vi "TPM with correction version 10-1-1 imaging_Min_20180112.vi"() -> ()   [LabVIEW 2018]
uses:
  Casao LabVIEW SDK 1.0.5/Haso/Data Haso/Wavefront parameters.ctl
  Casao LabVIEW SDK 1.0.5/Casao/Casao/Loop prefs.ctl
  Casao LabVIEW SDK 1.0.5/Haso/Data Haso/DataHaso.ctl
  <vilib>/Utility/file.llb/Read From Spreadsheet File (DBL).vi
  <vilib>/Utility/file.llb/Write To Spreadsheet File (DBL).vi
panel:
  in  "galvo phase":dbl=89.0
  out "output path":path
  out "Model Coefficients (µm) after":sgl[](array[numeric])
  out "Model Coefficients (µm) before":sgl[](array[numeric])
  in  "stop":bool
  out "Slice now":dbl
  in  "Iteration #":u16(ring)=1 items=["1"=1, "2"=2, "3"=3, "4"=4, "5"=5]
  in  "AO Exp Time":dbl(ring)=0.5 items=["0.2s"=0.2, "0.5s"=0.5, "1.0s"=1.0, "1.5s"=1.5]
  out "after correction":T1
  in  "Filter y tilt":bool=TRUE
  in  "Filter x tilt":bool=TRUE
  in  "Curvature filter":bool=TRUE
  out "PV":dbl
  out "RMS":dbl
  in  "Matrix path":path=path "C:/Documents and Settings/User/Desktop/zw/20160113 200nm bead command matrix.aomc"
  in  "Offset path":path=path "C:/Documents and Settings/User/Desktop/zw/2016-02-09 system resolution/100nm bead correction.dat"
  out "Camera image":u32[][](graph)
  out "RMS":dbl
  out "PV":dbl
  out "before correction":T1
  in  "Curvature filter":bool=TRUE
  in  "Filter y tilt":bool=TRUE
  in  "Filter x tilt":bool=TRUE
  out "after correction":dbl[][](graph) caption="Wavefront"
  out "before correction":dbl[][](graph) caption="Wavefront"
  in  "EMCCD ImExp Time (s)":dbl(ring)=0.5 items=["0.2"=0.2, "0.5"=0.5, "1.0"=1.0, "4.0"=4.0, "8.0"=8.0]
  in  "Step size(um)":dbl
  in  "Laser Power%(0-100)":dbl=10.0
  in  "Slices #":dbl=1.0
  in  "Average Frame #":dbl=10.0
  in  "Correction":bool
  # "OFF"
  # "ON"
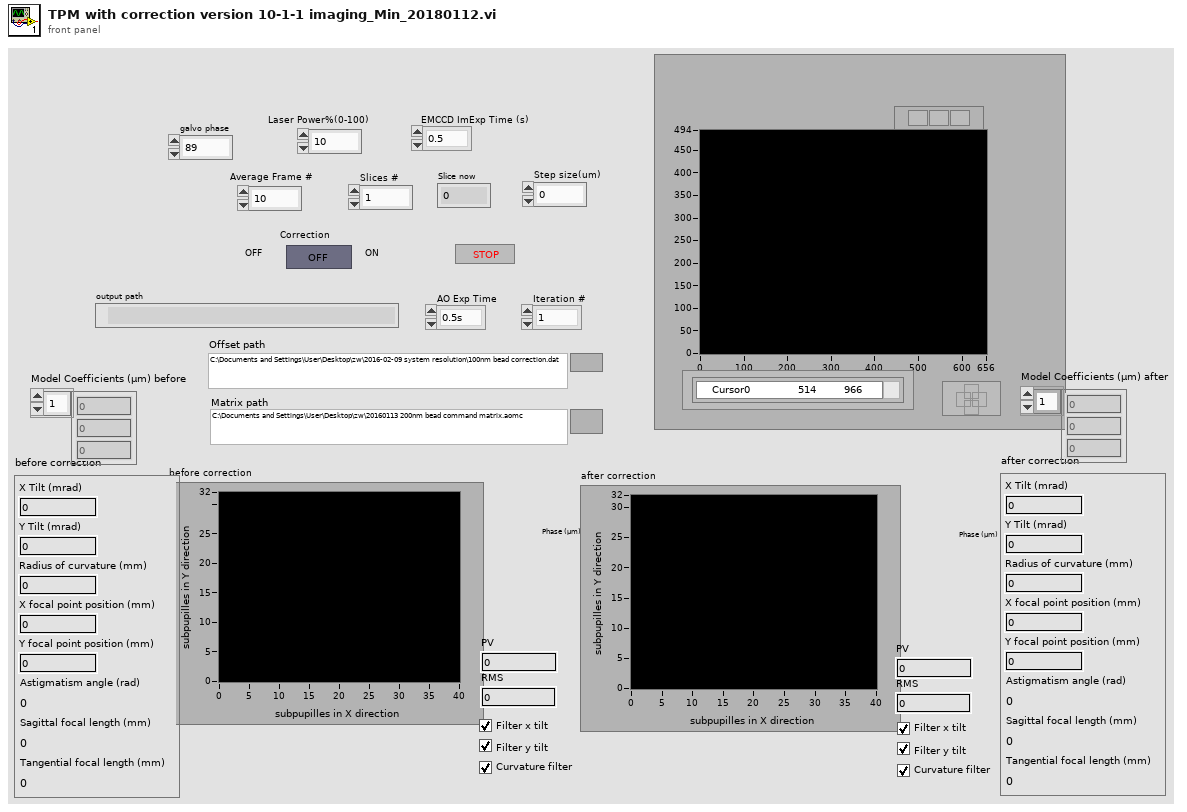
[diagram p1: front panel]
types:
  T1 = typedef "Wavefront parameters.ctl" = cluster{"X Tilt (mrad)":sgl, "Y Tilt (mrad)":sgl, "Radius of curvature (mm)":sgl, "X focal point position (mm)":sgl, "Y focal point position (mm)":sgl, "Astigmatism angle (rad)":sgl, "Sagittal focal length (mm)":sgl, "Tangential focal length (mm)":sgl}
  T2 = typedef "Loop prefs.ctl" = cluster{"Filter tilt on measurement (closed loop)":bool, "Correction gain (closed loop)":sgl, "Limit of subapertures off in CGP (%)":sgl, "Limit of saturated actuators (%)":sgl}
  T3 = cluster{"Filtre tilt X":bool, "Filtre tilt Y":bool, "Filtre courbure":bool}
  T4 = typedef "DataHaso.ctl" = i32
  T5 = cluster{"Measurement":T4, "Target":T4, "Manual target":T4}
  T6 = cluster{"Target for tilt":T4, "Target for focus":T4, "Target for all other aberrations":T4}
  T7 = typedef "Camera.ctl" = i32
  T8 = typedef "PhaseModul.ctl" = i32
  T9 = typedef "Haso.ctl" = i32
  T10 = typedef "Casao.ctl" = i32
  T11 = typedef "Image Compat.ctl" = cluster{"Signed/unsigned":bool, "Number of bits":T12, "Internal object id":i32, "Internal data id":i32}
  T12 = typedef "Data alignment enum.ctl" = enum16{"8", "16", "32"}
  T13 = typedef "Reconstruction prefs.ctl" = cluster{"Reconstruction type":enum16{"Modal", "Zonal"}, "Polynomial type":enum16{"Zernike", "Legendre"}, "Modal reconstruction prefs":T14, "Zonal reconstruction prefs":T17}
  T14 = typedef "Modal reconstruction prefs.ctl" = cluster{"Number of coefficients":u32, "Filtered coefficients":u32[], "RMS Zernike normalization":bool, "Matrix inversion method":u16, "Add zonal residual to modal fit ":bool, "Detection prefs":T15}
  T15 = typedef "PupilDetectionPrefs.ctl" = cluster{"Automatic pupil detection":bool, "Central occultation pupil":bool, "Semi-automatic pupil detection (find radius)":bool, "Semi-automatic pupil detection (find center)":bool, "Automatic pupil detection mode":enum16{"Contained", "Containing"}, "Start coordinates":cluster{"Pupil center (Zernike)":T16, "Pupil radius (Zernike)":sgl, "Pupil center (Legendre)":T16, "Pupil halfsize (Legendre)":T16}}
  T16 = typedef "Point2Df.ctl" = cluster{"X":sgl, "Y":sgl}
  T17 = typedef "Zonal reconstruction prefs.ctl" = cluster{"Number of weak iterations":u16, "Number of max iterations":u32, "Residual limit":sgl}
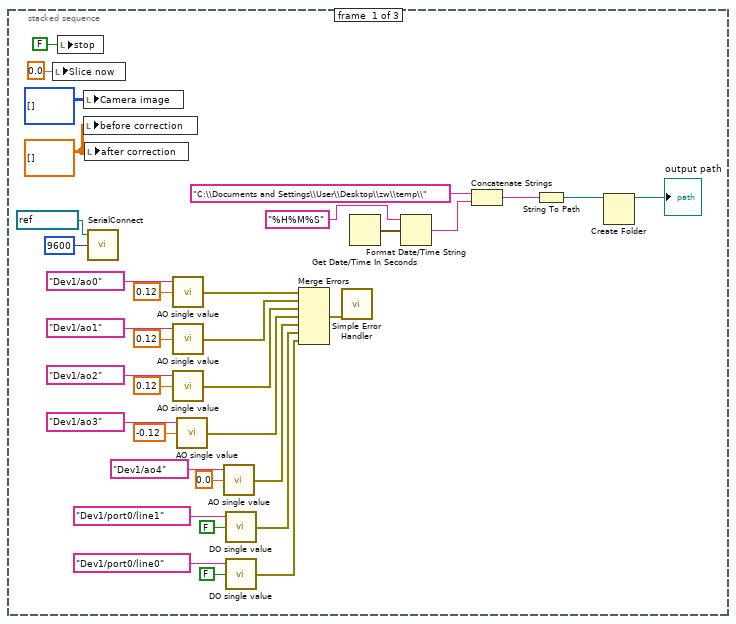
[diagram p2: hidden frame]
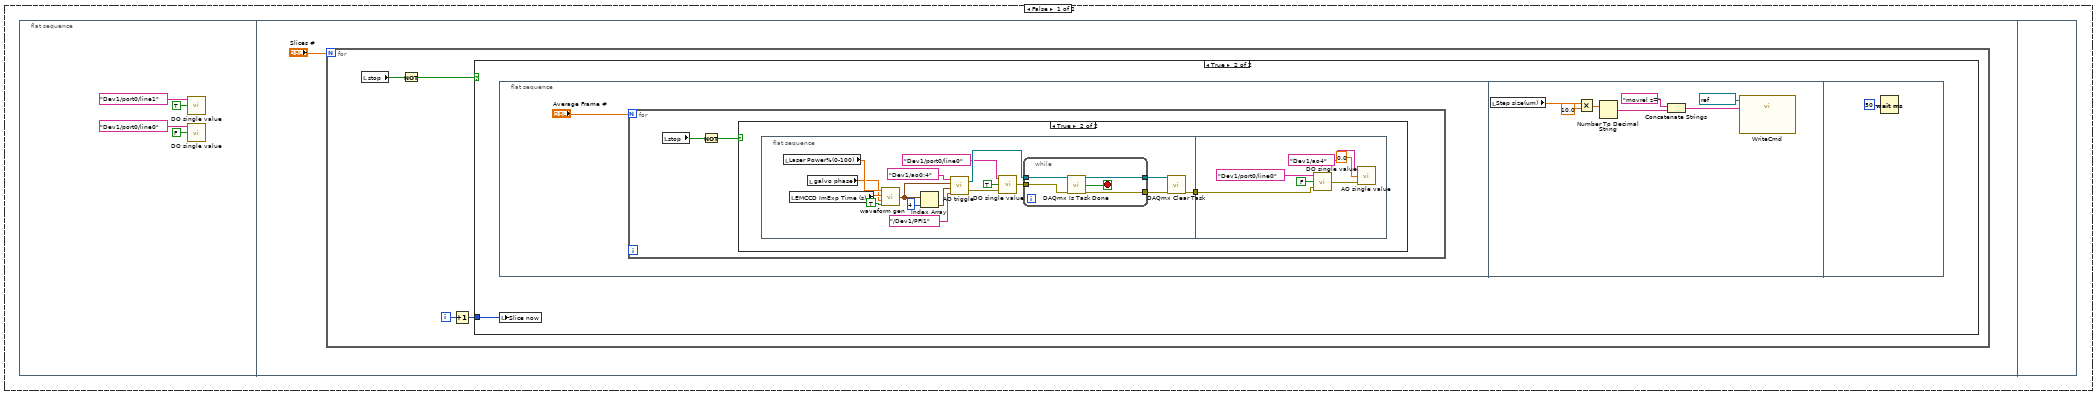
[diagram p3: hidden frame]
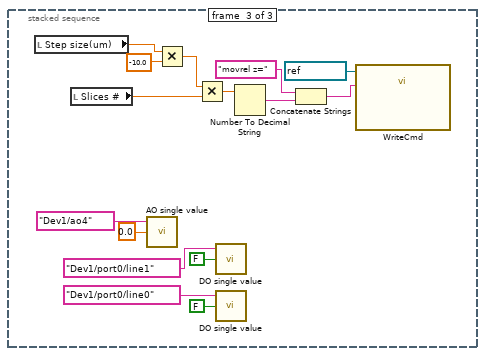
[diagram p10: hidden frame]
diagram:
  n1 = stacked-sequence {
    frame #0 {
      w34 = dbl[][] [] ("before correction")
      n2 = local write "Slice now"(0.0 ("Slice now")) -> ()
      n3 = local write "stop"(FALSE ("stop")) -> ()
      n4 = local write "Camera image"(u32[][] [] ("Camera image")) -> ()
      n5 = local write "before correction"(w34) -> ()
      n6 = local write "after correction"(w34) -> ()
      n7 = call "SerialConnect.vi"("baud rate (9600)"=u32 9600, "VISA resource name"=refnum<visa-resource-name> "COM1") -> ()  [unwired: 1 in, 3 out]
      n8 = call "AO single value.vi"("data"=0.12, "physical channels"=tag "Dev1/ao0") -> ("error out"=w17:errorcluster)  [unwired: 1 in]
      n9 = call "AO single value.vi"("data"=0.12, "physical channels"=tag "Dev1/ao1") -> ("error out"=w16:errorcluster)  [unwired: 1 in]
      n10 = call "AO single value.vi"("data"=0.12, "physical channels"=tag "Dev1/ao2") -> ("error out"=w15:errorcluster)  [unwired: 1 in]
      n11 = call "AO single value.vi"("data"=-0.12, "physical channels"=tag "Dev1/ao3") -> ("error out"=w14:errorcluster)  [unwired: 1 in]
      n12 = call "AO single value.vi"("data"=0.0, "physical channels"=tag "Dev1/ao4") -> ("error out"=w13:errorcluster)  [unwired: 1 in]
      n13 = call "DO single value.vi"("data"=FALSE, "lines"=tag "Dev1/port0/line1") -> ("error out"=w12:errorcluster)  [unwired: 1 in]
      n14 = call "DO single value.vi"("data"=FALSE, "lines"=tag "Dev1/port0/line0") -> ("error out"=w10:errorcluster)  [unwired: 1 in]
      n15 = Merge Errors(w17, w16, w15, w14, w13, w12, w10) -> (w11:errorcluster)
      n16 = call <vilib>:"Simple Error Handler.vi"("error in (no error)"=w11) -> ()  [unwired: 4 in, 5 out]
      n17 = Get Date/Time In Seconds() -> (seconds since 1Jan1904=w2:timestamp)
      n18 = Format Date/Time String(time format string (%c)="%H%M%S", seconds (now)=w2) -> (date/time string=w5:string)  [unwired: 1 in]
      n19 = Concatenate Strings("C:\\Documents and Settings\\User\\Desktop\\zw\\temp\\" ("string"), w5) -> (w6:string)
      n20 = String To Path(string=w6) -> (path=w7:path)
      n21 = Create Folder(path (use dialog)=w7) -> (created path=→"output path":path)  [unwired: 2 in, 2 out]
    }
    frame #1 {
      n22 = case shown="True" "Correction" {
        frame False {
          n23 = flat-sequence {
            frame #0 {
              n24 = call "DO single value.vi"("data"=TRUE, "lines"=tag "Dev1/port0/line1") -> ()  [unwired: 1 in, 1 out]
              n25 = call "DO single value.vi"("data"=FALSE, "lines"=tag "Dev1/port0/line0") -> ()  [unwired: 1 in, 1 out]
            }
            frame #1 {
              n26 = for {
                N: "Slices #" -> [_]
                i -> [w45]
                n27 = local read "stop"() -> (w43:bool)
                n28 = Not(x=w43) -> (.not. x?=w42:bool)
                n29 = Increment(x=w45) -> (x+1=w44:i32)
                n30 = case shown="True" w42 {
                  tunnel: w44 -> [_ w46]
                  frame False {
                  }
                  frame True {
                    n31 = local write "Slice now"(w46) -> ()
                    n32 = flat-sequence {
                      frame #0 {
                        n33 = for {
                          N: "Average Frame #" -> [_]
                          n34 = local read "stop"() -> (w48:bool)
                          n35 = Not(x=w48) -> (.not. x?=w49:bool)
                          n36 = case shown="True" w49 {
                            frame False {
                            }
                            frame True {
                              n37 = flat-sequence {
                                tunnel: [w52] -> w50
                                tunnel: w50 -> [w74]
                                frame #0 {
                                n38 = local read "Laser Power%(0-100)"() -> (w63:dbl)
                                n39 = local read "EMCCD ImExp Time (s)"() -> (w62:dbl)
                                n40 = local read "galvo phase"() -> (w51:dbl)
                                n41 = call "waveform gen.vi"("Boolean"=TRUE, "galvo phase"=w51, "Exposure Time (s)"=w62, "Laser Power%(0-100)"=w63) -> ("waveform"=w60:waveform(dbl)[])
                                n42 = Index Array(array=w60, index=4) -> (element=w61:waveform(dbl))
                                n43 = call "AO triggle.vi"("physical channels"=tag "Dev1/ao0:4", "data"=w60, "waveform"=w61, "trig source"=tag "/Dev1/PFI1") -> ("task out"=w57:refnum<k21>, "error out"=w54:errorcluster)  [unwired: 1 in]
                                n44 = call "DO single value.vi"("error in"=w54, "data"=TRUE, "lines"=tag "Dev1/port0/line0") -> ("error out"=w53:errorcluster)
                                n45 = while {
                                tunnel: [w72] -> w66
                                tunnel: [w71] -> w65
                                tunnel: w57 -> [w69]
                                tunnel: w53 -> [w68]
                                stop <- w70 stop-if-true
                                n46 = call <vilib>:"DAQmx Is Task Done.vi"("task/channels in"=w69, "error in"=w68) -> ("task out"=w72:refnum<k21>, "task done?"=w70:bool, "error out"=w71:errorcluster)  [unwired: 11 in]
                                }
                                n47 = call <vilib>:"DAQmx Clear Task.vi"("task in"=w66, "error in"=w65) -> ("error out"=w52:errorcluster)  [unwired: 13 in]
                                }
                                frame #1 {
                                n48 = call "DO single value.vi"("error in"=w74, "data"=FALSE, "lines"=tag "Dev1/port0/line0") -> ("error out"=w73:errorcluster)
                                n49 = call "AO single value.vi"("error in"=w73, "data"=0.0, "physical channels"=tag "Dev1/ao4") -> ()  [unwired: 1 out]
                                }
                              }
                            }
                          }
                        }
                      }
                      frame #1 {
                        n50 = local read "Step size(um)"() -> (w79:dbl)
                        n51 = Multiply(x=w79, y=10.0) -> (x*y=w81:dbl)
                        n52 = Number To Decimal String(number=w81) -> (decimal integer string=w84:string)  [unwired: 1 in]
                        n53 = Concatenate Strings("movrel z=", w84) -> (w83:string)
                        n54 = call "WriteCmd.vi"("Command"=w83, "VISA resource name"=refnum<visa-resource-name> "COM1") -> ()  [unwired: 1 in, 1 out]
                      }
                      frame #2 {
                        n55 = Wait (ms)(milliseconds to wait=u32 50) -> ()  [unwired: 1 out]
                      }
                    }
                  }
                }
              }
            }
            frame #2 {
            }
          }
        }
        frame True {
          n56 = flat-sequence {
            tunnel: [w102] -> w94
            tunnel: [w104] -> w93
            tunnel: [w103] -> w92
            tunnel: [w102] -> w91
            tunnel: [w101] -> w90
            tunnel: [w100] -> w88
            tunnel: [w95] -> w87
            tunnel: w94 -> [w123]
            tunnel: w93 -> [w122]
            tunnel: w92 -> [w121]
            tunnel: w91 -> [w118]
            tunnel: w90 -> [w117]
            tunnel: [w120] -> w89
            tunnel: w88 -> [w114]
            tunnel: w87 -> [w115]
            tunnel: w89 -> [w639]
            frame #0 {
              n57 = call "AO single value.vi"("data"=0.0, "physical channels"=tag "Dev1/ao4") -> ()  [unwired: 1 in, 1 out]
              n58 = local read "AO Exp Time"() -> (w105:dbl)
              n59 = call-poly <vilib>:"Read From Spreadsheet File.vi"("format (%.3f)"="%.8f", "file path (dialog if empty)"="Offset path") -> ("first row"=w95:dbl[])  [unwired: 5 in, 4 out]
              n60 = call "DO single value.vi"("data"=TRUE, "lines"=tag "Dev1/port0/line1") -> ()  [unwired: 1 in, 1 out]
              n61 = call "DO single value.vi"("data"=FALSE, "lines"=tag "Dev1/port0/line0") -> ()  [unwired: 1 in, 1 out]
              n62 = call "AO init.vi"("Exposure duration specified (s)"=w105, "Commands in"=w95, "Matrix path"="Matrix path") -> ("error out"=w102:errorcluster, "Camera"=w104:T7, "Mirror"=w100:T8, "Haso"=w103:T9, "Casao"=w101:T10)  [unwired: 3 in, 1 out]
            }
            frame #1 {
              n63 = call "Casao Set Preferences.vi"("error in (no error)"=w118, "Loop preferences"=T2 {"Filter tilt on measurement (closed loop)"=FALSE, "Correction gain (closed loop)"=0.75, "Limit of subapertures off in CGP (%)"=0.0, "Limit of saturated actuators (%)"=0.0}, "Casao"=w117) -> ("error out"=w112:errorcluster, "Casao (dup)"=w116:T10)  [unwired: 3 in]
              n64 = local read "Slices #"() -> (w124:dbl)
              n65 = call "PhaseModul apply command.vi"("error in (no error)"=w112, "Commands in"=w115, "Mirror"=w114) -> ("error out"=w111:errorcluster, "Mirror (dup)"=w113:T8)  [unwired: 2 in, 1 out]
              n66 = for {
                N: w124 -> [_]
                tunnel: w123 -> [w138]
                tunnel: w122 -> [w137]
                tunnel: w121 -> [w136]
                tunnel: w111 -> [w126]
                tunnel: [w135] -> w120
                tunnel: w113 -> [w127]
                tunnel: w116 -> [w134]
                tunnel: w115 -> [w125]
                i -> [w130]
                n67 = local read "stop"() -> (w132:bool)
                n68 = Increment(x=w130) -> (x+1=w133:i32)
                n69 = local write "Slice now"(w133) -> ()
                n70 = Not(x=w132) -> (.not. x?=w131:bool)
                n71 = case shown="True" w131 {
                  tunnel: w138 -> [_ w147]
                  tunnel: w137 -> [_ w146]
                  tunnel: w136 -> [_ w145]
                  tunnel: w126 -> [_ w144]
                  tunnel: [w139 w141] -> w135
                  tunnel: w127 -> [_ w143]
                  tunnel: w134 -> [w139 w142]
                  tunnel: w125 -> [_ w140]
                  frame False {
                  }
                  frame True {
                    n72 = flat-sequence {
                      tunnel: w147 -> [w187]
                      tunnel: w146 -> [w186]
                      tunnel: w145 -> [w185]
                      tunnel: w144 -> [w181]
                      tunnel: w143 -> [w172]
                      tunnel: w142 -> [w170]
                      tunnel: [w149] -> w141
                      tunnel: w140 -> [w148]
                      frame #0 {
                        n73 = flat-sequence {
                          tunnel: w170 -> [w190]
                          tunnel: w172 -> [w191]
                          tunnel: w181 -> [w192]
                          tunnel: w185 -> [w193]
                          tunnel: w186 -> [w194]
                          tunnel: w187 -> [w195]
                          tunnel: [w195] -> w155
                          tunnel: [w194] -> w154
                          tunnel: [w193] -> w153
                          tunnel: [w192] -> w152
                          tunnel: [w191] -> w151
                          tunnel: [w190] -> w150
                          tunnel: [w202] -> w161
                          tunnel: [w201] -> w160
                          tunnel: [w200] -> w159
                          tunnel: [w199] -> w158
                          tunnel: [w198] -> w157
                          tunnel: [w197] -> w156
                          tunnel: w155 -> [w202]
                          tunnel: w154 -> [w201]
                          tunnel: w153 -> [w200]
                          tunnel: w152 -> [w199]
                          tunnel: w151 -> [w198]
                          tunnel: w150 -> [w197]
                          tunnel: [w231] -> w184
                          tunnel: [w240] -> w183
                          tunnel: [w239] -> w182
                          tunnel: [w235] -> w180
                          tunnel: [w236] -> w179
                          tunnel: [w233] -> w173
                          tunnel: w161 -> [w232]
                          tunnel: w160 -> [w240]
                          tunnel: w159 -> [w239]
                          tunnel: w158 -> [w236]
                          tunnel: w157 -> [w234]
                          tunnel: w156 -> [w235]
                          tunnel: w148 -> [w230]
                          tunnel: w184 -> [w282]
                          tunnel: w183 -> [w281]
                          tunnel: w182 -> [w280]
                          tunnel: w180 -> [w279]
                          tunnel: w179 -> [w278]
                          tunnel: [w258] -> w178
                          tunnel: [w257] -> w177
                          tunnel: [w253] -> w176
                          tunnel: [w251] -> w175
                          tunnel: [w249] -> w174
                          tunnel: w173 -> [w244]
                          tunnel: [w243] -> w171
                          tunnel: [w241] -> w163
                          tunnel: w178 -> [w425]
                          tunnel: w177 -> [w424]
                          tunnel: w176 -> [w422]
                          tunnel: w175 -> [w421]
                          tunnel: w174 -> [w420]
                          tunnel: [w419] -> w169
                          tunnel: w171 -> [w418]
                          tunnel: [w417] -> w168
                          tunnel: [w416] -> w167
                          tunnel: [w415] -> w166
                          tunnel: [w414] -> w165
                          tunnel: [w413] -> w164
                          tunnel: w163 -> [w412]
                          tunnel: [w412] -> w162
                          tunnel: w169 -> [w604]
                          tunnel: w168 -> [w623]
                          tunnel: w167 -> [w622]
                          tunnel: w166 -> [w621]
                          tunnel: w165 -> [w611]
                          tunnel: w164 -> [w612]
                          tunnel: w162 -> [w610]
                          tunnel: [w604] -> w149
                          frame #0 {
                            n74 = call "AO single value.vi"("data"=-5.0, "physical channels"=tag "Dev1/ao5") -> ()  [unwired: 1 in, 1 out]
                          }
                          frame #1 {
                            n75 = local read "Average Frame #"() -> (w196:dbl)
                            n76 = for {
                              N: w196 -> [_]
                              n77 = local read "stop"() -> (w203:bool)
                              n78 = Not(x=w203) -> (.not. x?=w204:bool)
                              n79 = case shown="True" w204 {
                                frame False {
                                }
                                frame True {
                                n80 = flat-sequence {
                                frame #0 {
                                n81 = local read "Laser Power%(0-100)"() -> (w216:dbl)
                                n82 = local read "EMCCD ImExp Time (s)"() -> (w215:dbl)
                                n83 = call "waveform gen.vi"("Boolean"=TRUE, "galvo phase"="galvo phase", "Exposure Time (s)"=w215, "Laser Power%(0-100)"=w216) -> ("waveform"=w213:waveform(dbl)[])
                                n84 = Index Array(array=w213, index=4) -> (element=w214:waveform(dbl))
                                n85 = call "AO triggle.vi"("physical channels"=tag "Dev1/ao0:4", "data"=w213, "waveform"=w214, "trig source"=tag "/Dev1/PFI1") -> ("task out"=w210:refnum<k21>, "error out"=w207:errorcluster)  [unwired: 1 in]
                                n86 = call "DO single value.vi"("error in"=w207, "data"=TRUE, "lines"=tag "Dev1/port0/line0") -> ("error out"=w206:errorcluster)
                                n87 = while {
                                tunnel: [w225] -> w219
                                tunnel: [w224] -> w218
                                tunnel: w210 -> [w222]
                                tunnel: w206 -> [w221]
                                stop <- w223 stop-if-true
                                n88 = call <vilib>:"DAQmx Is Task Done.vi"("task/channels in"=w222, "error in"=w221) -> ("task out"=w225:refnum<k21>, "task done?"=w223:bool, "error out"=w224:errorcluster)  [unwired: 11 in]
                                }
                                n89 = call <vilib>:"DAQmx Clear Task.vi"("task in"=w219, "error in"=w218) -> ()  [unwired: 13 in, 1 out]
                                }
                                frame #1 {
                                n90 = call "AO single value.vi"("data"=0.0, "physical channels"=tag "Dev1/ao4") -> ()  [unwired: 1 in, 1 out]
                                n91 = call "DO single value.vi"("data"=FALSE, "lines"=tag "Dev1/port0/line0") -> ()  [unwired: 1 in, 1 out]
                                }
                                }
                                }
                              }
                            }
                          }
                          frame #2 {
                            n92 = call "PhaseModul apply command.vi"("error in (no error)"=w232, "Commands in"=w230, "Mirror"=w234) -> ("error out"=w231:errorcluster, "Mirror (dup)"=w233:T8)  [unwired: 2 in, 1 out]
                            n93 = call "AO single value.vi"("data"=1.0, "physical channels"=tag "Dev1/ao5") -> ()  [unwired: 1 in, 1 out]
                          }
                          frame #3 {
                            n94 = flat-sequence {
                              tunnel: [w291] -> w277
                              tunnel: [w290] -> w276
                              tunnel: [w289] -> w275
                              tunnel: [w288] -> w274
                              tunnel: [w287] -> w273
                              tunnel: w280 -> [w289]
                              tunnel: w281 -> [w290]
                              tunnel: w282 -> [w291]
                              tunnel: [w286] -> w272
                              tunnel: w279 -> [w286]
                              tunnel: [w285] -> w271
                              tunnel: w278 -> [w285]
                              tunnel: [w284] -> w245
                              tunnel: w244 -> [w284]
                              tunnel: w277 -> [w307]
                              tunnel: w276 -> [w308]
                              tunnel: w275 -> [w309]
                              tunnel: [w309] -> w270
                              tunnel: [w306] -> w269
                              tunnel: [w305] -> w268
                              tunnel: [w304] -> w267
                              tunnel: w274 -> [w304]
                              tunnel: [w303] -> w266
                              tunnel: w273 -> [w303]
                              tunnel: [w302] -> w265
                              tunnel: w272 -> [w302]
                              tunnel: [w301] -> w264
                              tunnel: w271 -> [w301]
                              tunnel: [w300] -> w246
                              tunnel: w245 -> [w300]
                              tunnel: w270 -> [w321]
                              tunnel: [w321] -> w261
                              tunnel: [w320] -> w262
                              tunnel: w269 -> [w320]
                              tunnel: [w319] -> w263
                              tunnel: w268 -> [w319]
                              tunnel: w267 -> [w314]
                              tunnel: w266 -> [w313]
                              tunnel: [w312] -> w260
                              tunnel: w265 -> [w312]
                              tunnel: [w311] -> w259
                              tunnel: w264 -> [w311]
                              tunnel: [w310] -> w247
                              tunnel: w246 -> [w310]
                              tunnel: w263 -> [w404]
                              tunnel: w262 -> [w364]
                              tunnel: w261 -> [w365]
                              tunnel: w260 -> [w390]
                              tunnel: w259 -> [w389]
                              tunnel: [w368] -> w256
                              tunnel: [w367] -> w255
                              tunnel: [w366] -> w254
                              tunnel: [w365] -> w252
                              tunnel: [w364] -> w250
                              tunnel: [w363] -> w248
                              tunnel: w247 -> [w362]
                              tunnel: [w362] -> w242
                              tunnel: [w336] -> w241
                              tunnel: [w410] -> w257
                              tunnel: [w411] -> w258
                              tunnel: w256 -> [w411]
                              tunnel: w255 -> [w410]
                              tunnel: w254 -> [w409]
                              tunnel: [w408] -> w253
                              tunnel: w252 -> [w408]
                              tunnel: [w407] -> w251
                              tunnel: w250 -> [w407]
                              tunnel: [w406] -> w249
                              tunnel: w248 -> [w406]
                              tunnel: [w405] -> w243
                              tunnel: w242 -> [w405]
                              frame #0 {
                                n95 = local read "Laser Power%(0-100)"() -> (w297:dbl)
                                n96 = local read "AO Exp Time"() -> (w296:dbl)
                                n97 = local read "galvo phase"() -> (w283:dbl)
                                n98 = call "waveform gen.vi"("Boolean"=FALSE, "galvo phase"=w283, "Exposure Time (s)"=w296, "Laser Power%(0-100)"=w297) -> ("waveform"=w295:waveform(dbl)[])
                                n99 = Index Array(array=w295, index=4) -> (element=w294:waveform(dbl))
                                n100 = call "AO triggle.vi"("physical channels"=tag "Dev1/ao0:4", "data"=w295, "waveform"=w294, "trig source"=tag "/Dev1/PFI1") -> ("task out"=w288:refnum<k21>, "error out"=w287:errorcluster)  [unwired: 1 in]
                              }
                              frame #1 {
                                n101 = call "Camera Start.vi"("error in (no error)"=w307, "camera"=w308) -> ("error out"=w305:errorcluster, "camera (dup)"=w306:T7)  [unwired: 4 in]
                              }
                              frame #2 {
                                n102 = while {
                                tunnel: [w327] -> w316
                                tunnel: [w326] -> w315
                                tunnel: w314 -> [w324]
                                tunnel: w313 -> [w323]
                                i -> [w322]
                                stop <- w325 stop-if-true
                                n103 = local write "Slice now"(w322) -> ()
                                n104 = call <vilib>:"DAQmx Is Task Done.vi"("task/channels in"=w324, "error in"=w323) -> ("task out"=w327:refnum<k21>, "task done?"=w325:bool, "error out"=w326:errorcluster)  [unwired: 11 in]
                                }
                                n105 = call "DO single value.vi"("data"=TRUE, "lines"=tag "Dev1/port0/line0") -> ()  [unwired: 1 in, 1 out]
                                n106 = call <vilib>:"DAQmx Clear Task.vi"("task in"=w316, "error in"=w315) -> ()  [unwired: 13 in, 1 out]
                              }
                              frame #3 {
                                n107 = call "Camera Get image.vi"("error in (no error)"=w404, "camera"=w364) -> ("error out"=w386:errorcluster, "Image"=w387:T11, "camera (dup)"=w388:T7)  [unwired: 3 in]
                                n108 = call "Camera Stop.vi"("error in (no error)"=w386, "camera"=w388) -> ()  [unwired: 4 in, 2 out]
                                n109 = call "Image get data.vi"("error in (no error)"=w386, "Image Compat"=w387) -> ("error out"=w376:errorcluster, "Array"=w385:u32[][], "Image Compat (dup)"=w375:T11)  [unwired: 3 in]
                                n110 = call "AO single value.vi"("data"=0.0, "physical channels"=tag "Dev1/ao4") -> ()  [unwired: 1 in, 1 out]
                                n111 = local write "Camera image"(w385) -> ()
                                n112 = call "Haso compute slopes.vi"("error in (no error)"=w376, "Image Compat"=w375, "Haso"=w365) -> ("error out"=w334:errorcluster, "Data Haso"=w338:T4)  [unwired: 1 in, 2 out]
                                n113 = call "DO single value.vi"("data"=FALSE, "lines"=tag "Dev1/port0/line0") -> ()  [unwired: 1 in, 1 out]
                                n114 = call "DataHaso ctor copie.vi"("error in (no error)"=w334, "DataHaso"=w338) -> ("error out"=w333:errorcluster, "new DataHaso"=w336:T4, "DataHaso (dup)"=w335:T4)  [unwired: 3 in]
                                n115 = call "DataHaso get reconstruction prefs.vi"("error in (no error)"=w333, "Data Haso"=w335) -> ("error out"=w349:errorcluster, "Reconstruction Preferences"=w345:T13, "Data Haso (dup)"=w348:T4)  [unwired: 3 in]
                                n116 = Bundle By Name(cluster=w345, "Reconstruction type"=enum16{"Modal", "Zonal"}."Modal", "Polynomial type"=enum16{"Zernike", "Legendre"}."Zernike", "Modal reconstruction prefs.Number of coefficients"=u32 32) -> (w344:T13)
                                n117 = call "DataHaso set reconstruction prefs.vi"("error in (no error)"=w349, "Reconstruction Preferences"=w344, "Data Haso"=w348) -> ("error out"=w346:errorcluster, "Data Haso (dup)"=w347:T4)  [unwired: 3 in]
                                n118 = call "DataHaso get modal coefficients.vi"("error in (no error)"=w346, "Data Haso"=w347) -> ("error out"=w339:errorcluster, "Coefficients (µm)"=w350:sgl[], "Data Haso (dup)"=w340:T4)  [unwired: 3 in]
                                "Model Coefficients (µm) before" <- w350
                                n119 = Bundle By Name(cluster=T3 {"Filtre tilt X"=FALSE, "Filtre tilt Y"=FALSE, "Filtre courbure"=FALSE} ("Filtre"), "Filtre tilt X"="Filter x tilt", "Filtre tilt Y"="Filter y tilt", "Filtre courbure"="Curvature filter") -> (w370:T3)
                                n120 = call "DataHaso parameters.vi"("error in (no error)"=w339, "Data Haso"=w340) -> ("error out"=w383:errorcluster, "Parameters"=w358:T1, "Data Haso (dup)"=w384:T4)  [unwired: 3 in]
                                "before correction" <- w358
                                n121 = control-ref of="before correction"() -> (w369:refnum<vi>)
                                n122 = call "DataHaso filter tilt or curvature.vi"("error in (no error)"=w383, "Filter (default: all true)"=w370, "Data Haso"=w384) -> ("error out"=w381:errorcluster, "Data Haso (dup)"=w382:T4)  [unwired: 3 in]
                                n123 = local read "Slice now"() -> (w352:dbl)
                                n124 = call "DataHaso phase.vi"("error in (no error)"=w381, "Data Haso"=w382) -> ("error out"=w379:errorcluster, "Phase (µm)"=w380:i32, "Data Haso (dup)"=w337:T4)  [unwired: 3 in]
                                n125 = Number To Decimal String(number=w352) -> (decimal integer string=w354:string)  [unwired: 1 in]
                                n126 = call "Formatter Intensity Graph.vi"("error in (no error)"=w379, "Intensity Graph"=w369, "Surface with pupil"=w380) -> ("error out"=w377:errorcluster, "Surface with pupil (dup)"=w378:i32)  [unwired: 2 in, 1 out]
                                n127 = call "Surface with pupil get stats.vi"("error in (no error)"=w377, "Surface Avec Pupille"=w378) -> ("error out"=w363:errorcluster, "PV"=w361:sgl, "RMS"=w360:dbl)  [unwired: 2 in, 1 out]
                                "PV" <- w361
                                "RMS" <- w360
                                n128 = local read "output path"() -> (w328:path)
                                n129 = Concatenate Strings("before_slice", w354, ".dat") -> (w329:string)
                                n130 = Cluster To Array(cluster=w358) -> (array=w359:sgl[])
                                n131 = Build Path(base path=w328, name or relative path=w329) -> (appended path=w330:path)
                                n132 = Build Array (concatenate)(w361, w360, w359, w350) -> (w357:dbl[])
                                n133 = Merge Errors(w363, w389) -> (w399:errorcluster)
                                n134 = Bundle By Name(cluster=T6 {"Target for tilt"=0, "Target for focus"=0, "Target for all other aberrations"=0} ("References"), "Target for tilt"=w336, "Target for focus"=w336) -> (w402:T6)
                                n135 = call "DataHaso ctor copie.vi"("error in (no error)"=w399, "DataHaso"=w337) -> ("error out"=w401:errorcluster, "new DataHaso"=w400:T4)  [unwired: 3 in, 1 out]
                                n136 = call-poly <vilib>:"Write To Spreadsheet File.vi"("transpose? (no:F)"=TRUE, "format (%.3f)"="%.6f", "1D data"=w357, "file path (dialog if empty)"=w330) -> ()  [unwired: 4 in, 1 out]
                                n137 = call "Casao Compute target.vi"("error in (no error)"=w401, "Targets"=w402, "DataHaso"=w400, "Casao"=w390) -> ("error out"=w397:errorcluster, "DataHaso (dup)"=w366:T4, "Casao (dup)"=w398:T10)  [unwired: 1 out]
                                n138 = Bundle By Name(cluster=T5 {"Measurement"=0, "Target"=0, "Manual target"=0} ("Slopes"), "Measurement"=w337, "Target"=w366) -> (w396:T5)
                                n139 = call "Casao get correction commands.vi"("Casao"=w398, "Slopes"=w396, "error in (no error)"=w397) -> ("Casao (dup)"=w368:T10, "Commands"=w393:sgl[], "error out"=w394:errorcluster)  [unwired: 2 in, 2 out]
                                n140 = call "PhaseModul apply command.vi"("error in (no error)"=w394, "Commands in"=w393, "Mirror"=w362) -> ("error out"=w367:errorcluster)  [unwired: 2 in, 2 out]
                              }
                              frame #4 {
                                n141 = call "DataHaso dtor.vi"("Data Haso"=w409) -> ()  [unwired: 6 in, 1 out]
                              }
                            }
                          }
                          frame #4 {
                            n142 = for {
                              N: "Iteration #" -> [_]
                              tunnel: w425 -> [w454]
                              tunnel: w424 -> [w453]
                              tunnel: w422 -> [w452]
                              tunnel: w421 -> [w451]
                              tunnel: w420 -> [w450]
                              tunnel: [w448] -> w419
                              tunnel: w418 -> [w443]
                              tunnel: [w442] -> w417
                              tunnel: [w440] -> w416
                              tunnel: [w438] -> w415
                              tunnel: [w436] -> w414
                              tunnel: [w433] -> w413
                              tunnel: w412 -> [w432]
                              i -> [w431]
                              n143 = Increment(x=w431) -> (x+1=w430:i32)
                              n144 = flat-sequence {
                                tunnel: [w479] -> w473
                                tunnel: [w480] -> w472
                                tunnel: [w481] -> w471
                                tunnel: [w485] -> w470
                                tunnel: [w484] -> w469
                                tunnel: [w483] -> w468
                                tunnel: [w482] -> w467
                                tunnel: w454 -> [w483]
                                tunnel: w453 -> [w482]
                                tunnel: w452 -> [w481]
                                tunnel: w451 -> [w480]
                                tunnel: w450 -> [w479]
                                tunnel: [w478] -> w444
                                tunnel: w443 -> [w478]
                                tunnel: w430 -> [w476]
                                tunnel: [w475] -> w427
                                tunnel: w473 -> [w502]
                                tunnel: w472 -> [w503]
                                tunnel: w471 -> [w504]
                                tunnel: [w504] -> w466
                                tunnel: [w501] -> w465
                                tunnel: [w500] -> w464
                                tunnel: [w499] -> w463
                                tunnel: w470 -> [w499]
                                tunnel: [w498] -> w462
                                tunnel: w469 -> [w498]
                                tunnel: [w497] -> w461
                                tunnel: w468 -> [w497]
                                tunnel: [w496] -> w460
                                tunnel: w467 -> [w496]
                                tunnel: [w495] -> w445
                                tunnel: w444 -> [w495]
                                tunnel: [w494] -> w428
                                tunnel: w427 -> [w494]
                                tunnel: w466 -> [w517]
                                tunnel: [w517] -> w457
                                tunnel: [w516] -> w458
                                tunnel: w465 -> [w516]
                                tunnel: [w515] -> w459
                                tunnel: w464 -> [w515]
                                tunnel: w463 -> [w510]
                                tunnel: w462 -> [w509]
                                tunnel: [w508] -> w456
                                tunnel: w461 -> [w508]
                                tunnel: [w507] -> w455
                                tunnel: w460 -> [w507]
                                tunnel: [w506] -> w446
                                tunnel: w445 -> [w506]
                                tunnel: [w505] -> w429
                                tunnel: w428 -> [w505]
                                tunnel: w459 -> [w585]
                                tunnel: w458 -> [w586]
                                tunnel: w457 -> [w587]
                                tunnel: w456 -> [w572]
                                tunnel: w455 -> [w571]
                                tunnel: [w551] -> w449
                                tunnel: [w550] -> w447
                                tunnel: w446 -> [w530]
                                tunnel: [w546] -> w441
                                tunnel: [w545] -> w439
                                tunnel: [w544] -> w437
                                tunnel: [w543] -> w435
                                tunnel: [w532] -> w434
                                tunnel: w432 -> [w529]
                                tunnel: w429 -> [w526]
                                tunnel: [w523] -> w426
                                tunnel: w449 -> [w599]
                                tunnel: [w598] -> w448
                                tunnel: w447 -> [w598]
                                tunnel: [w597] -> w442
                                tunnel: w441 -> [w597]
                                tunnel: [w596] -> w440
                                tunnel: w439 -> [w596]
                                tunnel: [w595] -> w438
                                tunnel: w437 -> [w595]
                                tunnel: [w591] -> w436
                                tunnel: w435 -> [w592]
                                tunnel: w434 -> [w594]
                                tunnel: [w594] -> w433
                                tunnel: w426 -> [w593]
                                frame #0 {
                                n145 = local read "Laser Power%(0-100)"() -> (w491:dbl)
                                n146 = local read "AO Exp Time"() -> (w490:dbl)
                                n147 = local read "galvo phase"() -> (w474:dbl)
                                n148 = call "waveform gen.vi"("Boolean"=FALSE, "galvo phase"=w474, "Exposure Time (s)"=w490, "Laser Power%(0-100)"=w491) -> ("waveform"=w489:waveform(dbl)[])
                                n149 = local read "Iteration #"() -> (w477:u16)
                                n150 = Index Array(array=w489, index=4) -> (element=w488:waveform(dbl))
                                n151 = Less?(x=w477, y=w476) -> (x < y?=w475:bool)
                                n152 = call "AO triggle.vi"("physical channels"=tag "Dev1/ao0:4", "data"=w489, "waveform"=w488, "trig source"=tag "/Dev1/PFI1") -> ("task out"=w485:refnum<k21>, "error out"=w484:errorcluster)  [unwired: 1 in]
                                }
                                frame #1 {
                                n153 = call "Camera Start.vi"("error in (no error)"=w502, "camera"=w503) -> ("error out"=w500:errorcluster, "camera (dup)"=w501:T7)  [unwired: 4 in]
                                }
                                frame #2 {
                                n154 = while {
                                tunnel: [w522] -> w512
                                tunnel: [w521] -> w511
                                tunnel: w510 -> [w519]
                                tunnel: w509 -> [w518]
                                stop <- w520 stop-if-true
                                n155 = call <vilib>:"DAQmx Is Task Done.vi"("task/channels in"=w519, "error in"=w518) -> ("task out"=w522:refnum<k21>, "task done?"=w520:bool, "error out"=w521:errorcluster)  [unwired: 11 in]
                                }
                                n156 = call "DO single value.vi"("data"=TRUE, "lines"=tag "Dev1/port0/line0") -> ()  [unwired: 1 in, 1 out]
                                n157 = call <vilib>:"DAQmx Clear Task.vi"("task in"=w512, "error in"=w511) -> ()  [unwired: 13 in, 1 out]
                                }
                                frame #3 {
                                n158 = call "Camera Get image.vi"("error in (no error)"=w585, "camera"=w586) -> ("error out"=w568:errorcluster, "Image"=w569:T11, "camera (dup)"=w570:T7)  [unwired: 3 in]
                                n159 = call "Camera Stop.vi"("error in (no error)"=w568, "camera"=w570) -> ()  [unwired: 4 in, 2 out]
                                n160 = call "Image get data.vi"("error in (no error)"=w568, "Image Compat"=w569) -> ("error out"=w558:errorcluster, "Array"=w567:u32[][], "Image Compat (dup)"=w557:T11)  [unwired: 3 in]
                                n161 = call "AO single value.vi"("data"=0.0, "physical channels"=tag "Dev1/ao4") -> ()  [unwired: 1 in, 1 out]
                                n162 = local write "Camera image"(w567) -> ()
                                n163 = call "Haso compute slopes.vi"("error in (no error)"=w558, "Image Compat"=w557, "Haso"=w587) -> ("error out"=w535:errorcluster, "Data Haso"=w534:T4)  [unwired: 1 in, 2 out]
                                n164 = call "DO single value.vi"("data"=FALSE, "lines"=tag "Dev1/port0/line0") -> ()  [unwired: 1 in, 1 out]
                                n165 = call "DataHaso get reconstruction prefs.vi"("error in (no error)"=w535, "Data Haso"=w534) -> ("error out"=w541:errorcluster, "Reconstruction Preferences"=w540:T13, "Data Haso (dup)"=w542:T4)  [unwired: 3 in]
                                n166 = Bundle By Name(cluster=w540, "Reconstruction type"=enum16{"Modal", "Zonal"}."Modal", "Polynomial type"=enum16{"Zernike", "Legendre"}."Zernike", "Modal reconstruction prefs.Number of coefficients"=u32 32) -> (w539:T13)
                                n167 = call "DataHaso set reconstruction prefs.vi"("error in (no error)"=w541, "Reconstruction Preferences"=w539, "Data Haso"=w542) -> ("error out"=w527:errorcluster, "Data Haso (dup)"=w528:T4)  [unwired: 3 in]
                                n168 = call "DataHaso get modal coefficients.vi"("error in (no error)"=w527, "Data Haso"=w528) -> ("error out"=w533:errorcluster, "Coefficients (µm)"=w532:sgl[], "Data Haso (dup)"=w531:T4)  [unwired: 3 in]
                                "Model Coefficients (µm) after" <- w532
                                n169 = Bundle By Name(cluster=T3 {"Filtre tilt X"=FALSE, "Filtre tilt Y"=FALSE, "Filtre courbure"=FALSE} ("Filtre"), "Filtre tilt X"="Filter x tilt", "Filtre tilt Y"="Filter y tilt", "Filtre courbure"="Curvature filter") -> (w555:T3)
                                n170 = call "DataHaso parameters.vi"("error in (no error)"=w533, "Data Haso"=w531) -> ("error out"=w565:errorcluster, "Parameters"=w544:T1, "Data Haso (dup)"=w566:T4)  [unwired: 3 in]
                                "after correction" <- w544
                                n171 = control-ref of="after correction"() -> (w549:refnum<vi>)
                                n172 = call "DataHaso filter tilt or curvature.vi"("error in (no error)"=w565, "Filter (default: all true)"=w555, "Data Haso"=w566) -> ("error out"=w563:errorcluster, "Data Haso (dup)"=w564:T4)  [unwired: 3 in]
                                n173 = call "DataHaso phase.vi"("error in (no error)"=w563, "Data Haso"=w564) -> ("error out"=w561:errorcluster, "Phase (µm)"=w562:i32, "Data Haso (dup)"=w548:T4)  [unwired: 3 in]
                                n174 = call "Formatter Intensity Graph.vi"("error in (no error)"=w561, "Intensity Graph"=w549, "Surface with pupil"=w562) -> ("error out"=w559:errorcluster, "Surface with pupil (dup)"=w560:i32)  [unwired: 2 in, 1 out]
                                n175 = call "Surface with pupil get stats.vi"("error in (no error)"=w559, "Surface Avec Pupille"=w560) -> ("error out"=w580:errorcluster, "PV"=w545:sgl, "RMS"=w546:dbl)  [unwired: 2 in, 1 out]
                                "RMS" <- w546
                                "PV" <- w545
                                n176 = Merge Errors(w580, w571) -> (w579:errorcluster)
                                n177 = Bundle By Name(cluster=T6 {"Target for tilt"=0, "Target for focus"=0, "Target for all other aberrations"=0} ("References"), "Target for tilt"=w529, "Target for focus"=w529) -> (w583:T6)
                                n178 = call "DataHaso ctor copie.vi"("error in (no error)"=w579, "DataHaso"=w548) -> ("error out"=w582:errorcluster, "new DataHaso"=w581:T4, "DataHaso (dup)"=w547:T4)  [unwired: 3 in]
                                n179 = call "Casao Compute target.vi"("error in (no error)"=w582, "Targets"=w583, "DataHaso"=w581, "Casao"=w572) -> ("error out"=w577:errorcluster, "DataHaso (dup)"=w551:T4, "Casao (dup)"=w578:T10)  [unwired: 1 out]
                                n180 = Bundle By Name(cluster=T5 {"Measurement"=0, "Target"=0, "Manual target"=0} ("Slopes"), "Measurement"=w547, "Target"=w551) -> (w576:T5)
                                n181 = call "Casao get correction commands.vi"("Casao"=w578, "Slopes"=w576, "error in (no error)"=w577) -> ("Casao (dup)"=w550:T10, "Commands"=w543:sgl[], "error out"=w523:errorcluster)  [unwired: 2 in, 2 out]
                                n182 = case shown="True" w526 {
                                tunnel: w523 -> [_ w590]
                                tunnel: w543 -> [_ w589]
                                tunnel: w530 -> [_ w588]
                                frame False {
                                }
                                frame True {
                                n183 = call "PhaseModul apply command.vi"("error in (no error)"=w590, "Commands in"=w589, "Mirror"=w588) -> ()  [unwired: 2 in, 3 out]
                                }
                                }
                                }
                                frame #4 {
                                n184 = call "DataHaso dtor.vi"("Data Haso"=w599) -> ()  [unwired: 6 in, 1 out]
                                n185 = case shown="Error" w593 {
                                tunnel: w592 -> [w600 _]
                                tunnel: [w600 w601] -> w591
                                frame No Error {
                                }
                                frame Error {
                                n186 = Initialize Array(0.0 ("element"), 52 ("dimension size")) -> (w601:dbl[])
                                }
                                }
                                }
                              }
                            }
                          }
                          frame #5 {
                            n187 = call "DataHaso dtor.vi"("Data Haso"=w610) -> ()  [unwired: 6 in, 1 out]
                            n188 = local read "Slice now"() -> (w615:dbl)
                            n189 = Cluster To Array(cluster=w621) -> (array=w620:sgl[])
                            n190 = Build Array (concatenate)(w622, w623, w620, w612) -> (w628:dbl[])
                            n191 = Number To Decimal String(number=w615) -> (decimal integer string=w625:string)  [unwired: 1 in]
                            n192 = Number To Decimal String(number=w615) -> (decimal integer string=w617:string)  [unwired: 1 in]
                            n193 = call "AO single value.vi"("data"=0.0, "physical channels"=tag "Dev1/ao4") -> ()  [unwired: 1 in, 1 out]
                            n194 = local read "output path"() -> (w605:path)
                            n195 = Concatenate Strings("afterC_slice", w625, ".dat") -> (w609:string)
                            n196 = Concatenate Strings("command", w617, ".dat") -> (w606:string)
                            n197 = Build Path(base path=w605, name or relative path=w609) -> (appended path=w608:path)
                            n198 = Build Path(base path=w605, name or relative path=w606) -> (appended path=w607:path)
                            n199 = call-poly <vilib>:"Write To Spreadsheet File.vi"("transpose? (no:F)"=TRUE, "format (%.3f)"="%.6f", "1D data"=w628, "file path (dialog if empty)"=w608) -> ()  [unwired: 4 in, 1 out]
                            n200 = call-poly <vilib>:"Write To Spreadsheet File.vi"("transpose? (no:F)"=TRUE, "format (%.3f)"="%.6f", "1D data"=w611, "file path (dialog if empty)"=w607) -> ()  [unwired: 4 in, 1 out]
                          }
                          frame #6 {
                            n201 = local read "Step size(um)"() -> (w637:dbl)
                            n202 = Multiply(x=w637, y=10.0) -> (x*y=w635:dbl)
                            n203 = Number To Decimal String(number=w635) -> (decimal integer string=w632:string)  [unwired: 1 in]
                            n204 = Concatenate Strings("movrel z=", w632) -> (w633:string)
                            n205 = call "WriteCmd.vi"("Command"=w633, "VISA resource name"=refnum<visa-resource-name> "COM1") -> ()  [unwired: 1 in, 1 out]
                          }
                          frame #7 {
                            n206 = Wait (ms)(milliseconds to wait=u32 50) -> ()  [unwired: 1 out]
                          }
                        }
                      }
                    }
                  }
                }
                n207 = call "AO single value.vi"("data"=0.0, "physical channels"=tag "Dev1/ao4") -> ()  [unwired: 1 in, 1 out]
              }
            }
            frame #2 {
              n208 = call "Casao dtor.vi"("Casao"=w639) -> ()  [unwired: 6 in, 1 out]
            }
          }
        }
      }
    }
    frame #2 {
      n209 = local read "Step size(um)"() -> (w647:dbl)
      n210 = local read "Slices #"() -> (w640:dbl)
      n211 = call "AO single value.vi"("data"=0.0, "physical channels"=tag "Dev1/ao4") -> ()  [unwired: 1 in, 1 out]
      n212 = Multiply(x=w647, y=-10.0) -> (x*y=w648:dbl)
      n213 = Multiply(x=w648, y=w640) -> (x*y=w646:dbl)
      n214 = call "DO single value.vi"("data"=FALSE, "lines"=tag "Dev1/port0/line1") -> ()  [unwired: 1 in, 1 out]
      n215 = call "DO single value.vi"("data"=FALSE, "lines"=tag "Dev1/port0/line0") -> ()  [unwired: 1 in, 1 out]
      n216 = Number To Decimal String(number=w646) -> (decimal integer string=w642:string)  [unwired: 1 in]
      n217 = Concatenate Strings("movrel z=", w642) -> (w643:string)
      n218 = call "WriteCmd.vi"("Command"=w643, "VISA resource name"=refnum<visa-resource-name> "COM1") -> ()  [unwired: 1 in, 1 out]
    }
  }
